vi "Check for Viewer Requests.vi"(8 "error in":errorcluster, 11 "data server thread in":refnum<class "Data Server Thread.lvclass">) -> (0 "error out":errorcluster, 3 "data server thread out":refnum<class "Data Server Thread.lvclass">)   [LabVIEW 2020, in "DSF Core.lvlib" / "Data Server Thread.lvclass"]
uses:
  Data Server Thread.lvclass
  Data Server Thread.lvclass/Data Server Thread.ctl
  Transfer/Transfer.lvclass/Transfer.ctl
  Buffers/Buffers.lvclass/Buffers.ctl
  <vilib>/NI/Memory Manager/Classes/Pointer/Pointer.lvclass/Pointer.ctl
  <vilib>/NI/Memory Manager/Classes/Pointer/Subset.vi
  Buffers/Get Active Buffers.vi
  <vilib>/NI/Memory Manager/Classes/Pointer/Get Address.vi
  <vilib>/NI/Memory Manager/Classes/Pointer/Encapsulate.vi
  <vilib>/NI/Memory Manager/Classes/Pointer/Check Null Pointer.vi
  <vilib>/NI/Memory Manager/Classes/Pointer/Check Length.vi
  <vilib>/NI/Memory Manager/Classes/Pointer/Set Size.vi
  <vilib>/NI/Memory Manager/Classes/Pointer/Set Address.vi
  <vilib>/NI/Memory Manager/Classes/Pointer/Set Internal.vi
  <vilib>/NI/Memory Manager/Classes/Pointer/Errors.vi
  <vilib>/NI/Memory Manager/Classes/Pointer/Null Pointer.vi
  <vilib>/NI/Memory Manager/Classes/Pointer/Is Null.vi
  <vilib>/NI/Memory Manager/Classes/Pointer/Get Size.vi
  <vilib>/NI/Memory Manager/Classes/Pointer/Check Bounds (Pointer).vi
  <vilib>/NI/Memory Manager/Classes/Pointer/Create Error.vi
  <vilib>/NI/Memory Manager/Classes/Pointer/Out of Bounds.vi
  <vilib>/NI/Memory Manager/VIs/New Error Cluster.vi
  <vilib>/NI/Memory Manager/VIs/New Error Cluster (512B).vi
  <vilib>/NI/Memory Manager/VIs/Set Error Status.vi
  <vilib>/NI/Memory Manager/VIs/Set Error Code.vi
  <vilib>/NI/Memory Manager/VIs/Set Error Source.vi
  <vilib>/NI/Memory Manager/Constants/Constants.vi
  <vilib>/NI/Memory Manager/Constants/Library Name.vi
  <vilib>/NI/Memory Manager/Classes/Pointer/Pointer Error Info.vi
  <vilib>/NI/Memory Manager/VIs/Write String to Source.vi
  <vilib>/NI/Memory Manager/Constants/Pointer Class Name.vi
  <vilib>/NI/Memory Manager/Classes/Pointer/Write Pointer Size to Error.vi
  <vilib>/NI/Memory Manager/VIs/Write Numeric to Source.vi
  <vilib>/NI/Memory Manager/VIs/Write Numeric Scalar to Source (Base10 U64).vi
  Buffer/Buffer.lvclass
  C:/Program Files (x86)/National Instruments/LabVIEW 2020/vi.lib/NI/Memory Manager/Classes/Pointer/Pointer.lvclass
  Status/Status Pointer.lvclass
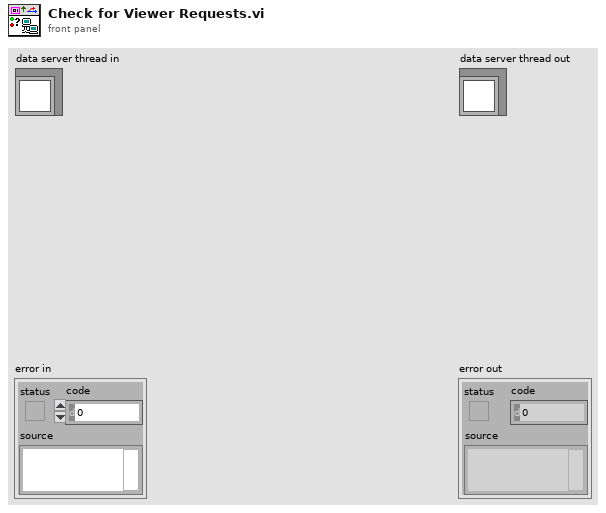
[diagram p1: front panel]
types:
  T1 = typedef "DSF Core.lvlib/Data Server Thread.lvclass/Framework.ctl" = cluster{"Framework Status":refnum<class "Status Pointer.lvclass">, "Plugins":T2[]}
  T2 = typedef "DSF Core.lvlib/Data Server Thread.lvclass/Plugin.ctl" = cluster{"Plugin Status":refnum<class "Status Pointer.lvclass">, "Groups":T3[]}
  T3 = typedef "DSF Core.lvlib/Data Server Thread.lvclass/Group.ctl" = cluster{"Group Buffers":refnum<class "Buffers.lvclass">, "Group Status":refnum<class "Status Pointer.lvclass">, "Transfers":refnum<class "Transfer.lvclass">[]}
  T4 = typedef "DSF Core.lvlib/Data Server Thread.lvclass/Viewer Data.ctl" = cluster{"remote address":string, "remote port":u16, "connection ID":refnum<k5>, "Buffer":refnum<class "Buffer.lvclass">, "Status":refnum<class "Status Pointer.lvclass">}
  T5 = typedef "DSF Core.lvlib/DSF Buffer Subset Descriptor.ctl" = cluster{"buffer type":T6, "plugin id":i32, "group id":i32, "transfer id":i32, "offset":u64, "length":i64}
  T6 = typedef "DSF Core.lvlib/DSF Buffer Type.ctl" = enum16{"Engine", "String"}
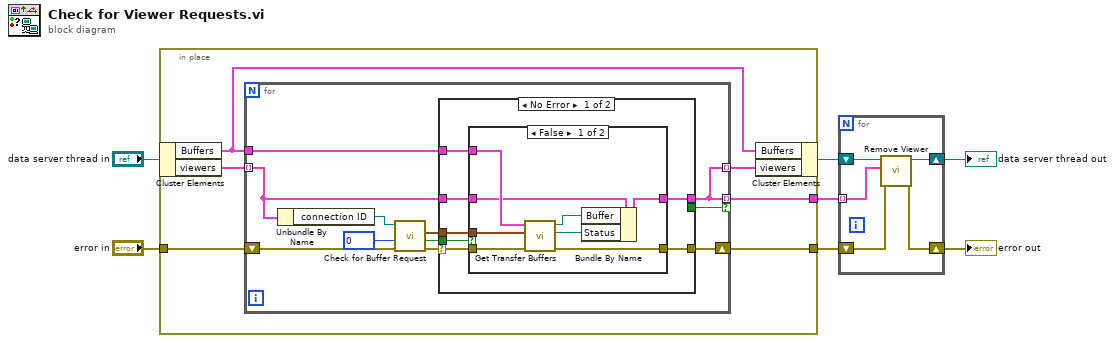
[diagram p0: block diagram]
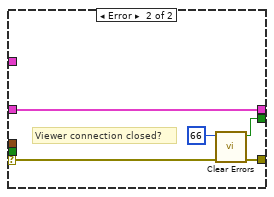
[diagram p3: hidden frame]
diagram:
  n1 = in-place {
    in-place-border: [w13] -> w4
    in-place-border: "error in" -> [w12]
    in-place-border: [w8] -> w1
    n2 = in-place-cluster #1("data server thread in") -> ("Buffers"=w9:T1, "viewers"=w11:T4[])
    n3 = for {
      tunnel: w11 -> [w21] mode=indexing
      shift-right: [w19] -> w13
      shift-left: w12 -> [w24]
      tunnel: [w14] -> w10 mode=indexing
      tunnel: w9 -> [w17]
      tunnel: [w14] -> w8 mode=indexing if=w16
      n4 = Unbundle By Name(w21) -> ("connection ID"=w23:refnum<k5>)
      n5 = call "Check for Buffer Request.vi"("error in (no error)"=w24, "timeout ms (25000)"=0, "connection ID in"=w23) -> ("error out"=w15:errorcluster, "timed out?"=w20:bool, "buffer descriptor"=w18:T5)  [unwired: 5 in, 1 out]
      n6 = case shown="No Error" w15 {
        selector: w15 -> [w25 w45]
        tunnel: w21 -> [w31 w46]
        tunnel: w20 -> [w30 _]
        tunnel: [w29 w46] -> w14
        tunnel: [w28 w43] -> w19
        tunnel: w18 -> [w27 _]
        tunnel: w17 -> [w26 _]
        tunnel: [_ w42] -> w16
        frame No Error {
          n7 = case shown="False" w30 {
            tunnel: w31 -> [w33 w40]
            tunnel: w27 -> [w34 _]
            tunnel: [w39 w40] -> w29
            tunnel: w25 -> [w35 w41]
            tunnel: [w36 w41] -> w28
            tunnel: w26 -> [w38 _]
            frame False {
              n8 = call "Get Transfer Buffers.vi"("error in"=w35, "buffer descriptor"=w34, "buffers"=w38) -> ("error out"=w36:errorcluster, "status"=w32:refnum<class "Status Pointer.lvclass">, "buffer"=w37:refnum<class "Buffer.lvclass">)  [unwired: 6 in]
              n9 = Bundle By Name(cluster=w33, "Buffer"=w37, "Status"=w32) -> (w39:T4)
            }
            frame True {
            }
          }
        }
        frame Error {
          # "Viewer connection closed?"
          n10 = call <vilib>:"Clear Errors.vi"("error in (no error)"=w45, "specific error code to clear (0: all)"=66) -> ("error out"=w43:errorcluster, "specific error cleared?"=w42:bool)  [unwired: 4 in]
        }
      }
    }
    n11 = in-place-cluster #1("Buffers"=w9, "viewers"=w10) -> (w5:refnum<class "Data Server Thread.lvclass">)
  }
  n12 = for {
    shift-right: [w50] -> w3
    shift-left: w5 -> [w51]
    shift-right: [w48] -> w2
    shift-left: w4 -> [w49]
    tunnel: w1 -> [w47] mode=indexing
    n13 = call "Remove Viewer.vi"("error in"=w49, "viewer"=w47, "Data Server Thread in"=w51) -> ("error out"=w48:errorcluster, "Data Server Thread out"=w50:refnum<class "Data Server Thread.lvclass">)  [unwired: 7 in]
  }
  "error out" <- w2
  "data server thread out" <- w3
